vi "Close Launcher.vi"(8 "error in (no error)":errorcluster, 11 "Actor wLauncher in":refnum<class "Actor wLauncher.lvclass">) -> (0 "error out":errorcluster, 3 "Actor wLauncher out":refnum<class "Actor wLauncher.lvclass">)   [LabVIEW 2017, in "Framework.lvlib" / "Actor wLauncher.lvclass"]
uses:
  Actor wLauncher.lvclass
  Actor wLauncher.lvclass/Actor wLauncher.ctl
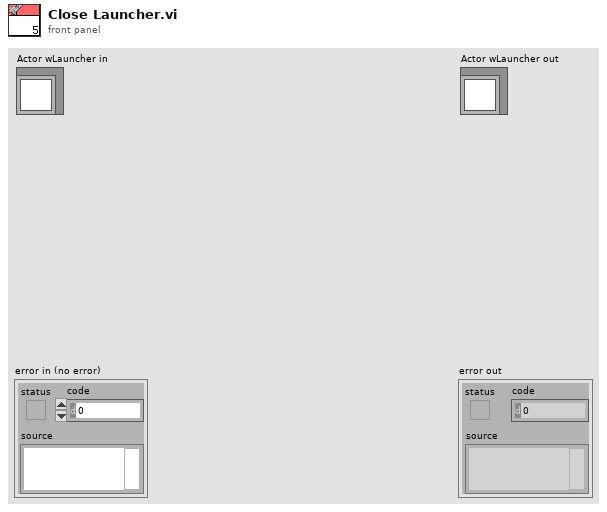
[diagram p1: front panel]
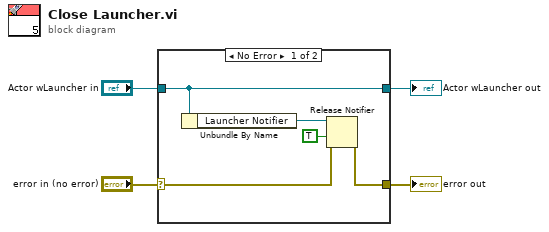
[diagram p0: block diagram]
diagram:
  n1 = case shown="No Error" "error in (no error)" {
    selector: "error in (no error)" -> [w7 w11]
    tunnel: [w6 w11] -> w3
    tunnel: [w9 w10] -> w1
    tunnel: "Actor wLauncher in" -> [w9 w10]
    frame No Error {
      n2 = Unbundle By Name(w9) -> ("Launcher Notifier"=w8:refnum<notifier>)
      n3 = Release Notifier(notifier=w8, force destroy? (F)=TRUE, error in (no error)=w7) -> (error out=w6:errorcluster)  [unwired: 2 out]
    }
    frame Error {
    }
  }
  "error out" <- w3
  "Actor wLauncher out" <- w1
